vi "Read distance_deg.vi"(8 "error in (no error)":errorcluster, 11 "SunMoonStatus in":refnum<class "SunMoonStatus.lvclass">) -> (0 "error out":errorcluster, 2 "distance_deg":dbl[unit], 3 "SunMoonStatus out":refnum<class "SunMoonStatus.lvclass">)   [LabVIEW 2014, in "TCSDataDefinitions.lvlib" / "TCSPublicStatus.lvlib" / "Limits.lvlib" / "SunMoonStatus.lvclass"]
uses:
  SunMoonStatus.lvclass
  SunMoonStatus.lvclass/SunMoonStatus.ctl
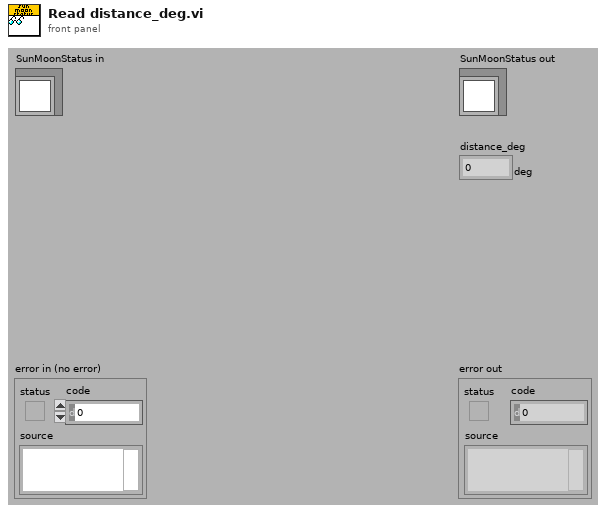
[diagram p1: front panel]
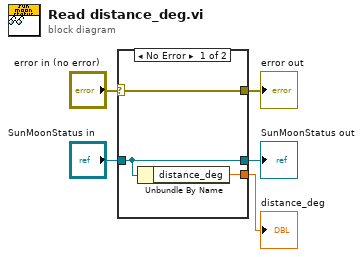
[diagram p0: block diagram]
diagram:
  n1 = case shown="No Error" "error in (no error)" {
    selector: "error in (no error)" -> [w8 w9]
    tunnel: [w8 w9] -> w4
    tunnel: [w7 w10] -> w2
    tunnel: "SunMoonStatus in" -> [w7 w10]
    tunnel: [w6 _] -> w1
    frame No Error {
      n2 = Unbundle By Name(w7) -> ("distance_deg"=w6:dbl[unit])
    }
    frame Error {
    }
  }
  "error out" <- w4
  "SunMoonStatus out" <- w2
  "distance_deg" <- w1
